vi "Demo1_Filter.vi"(11 "input data":fxp<+/-,16,1>) -> (3 "output data":fxp<+/-,16,2>)   [LabVIEW 2023]
doc: "----------------------\n\nThis filter is configured as follows:\n\n<b>Filter Configuration</b>\nType: Single Rate\nStructure: FIR Direct Form\n\n<b>Input Data Type</b>\nType: fixed-point <±,16,1> [-1.000000E+0,9.999695E-1]:3.051758E-5\n\n<b>Output Data Type</b>\nType: fixed-point <±,16,2> [-2.000000E+0,1.999939E+0]:6.103516E-5\nRounding mode: Truncate\nOverflow mode: Wrap\n\n<b>Implementation</b>\nNumber of channels: 1\nMaximum input sampling rate per channel @ 40MHz: 754.717kHz\nGain processing: On Target\nMethod: Multiple Multiply-Accumulator\nNumber of multiply pipeline stages: 1\n\n<b>Execution Mode</b>\nOutside single-cycle Timed Loop\nThroughput: 53 cycles/sample\n\n<b>Estimated Resources</b>\nNumber of multiply-accumulate units: 1\nMultiply operation: 16bits x 16bits => 32bits"
uses:
  <vilib>/Platform/TimedLoop/XDataNode/timing_clust.ctl
  <vilib>/Platform/TimedLoop/XDataNode/nitl_modes.ctl
  <vilib>/Platform/TimedLoop/XDataNode/wakeup.ctl
  <vilib>/Platform/TimedLoop/XDataNode/XDataNode.xnode
  <vilib>/Platform/TimedLoop/XDataNode/XDNodeRunTimeDep.lvlib
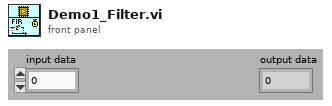
[diagram p1: front panel]
types:
  T1 = typedef "XDNodeRunTimeDep.lvlib/timing_clust.ctl" = cluster{"Expected End [f-1]":u64, "Actual End [f-1]":u64, "Finished Late? [f-1]":bool, "Expected End [i-1]":u64, "Actual End [i-1]":u64, "Finished Late? [i-1]":bool, "Expected Start [i]":u64, "Actual Start [i]":u64, "Expected Start [f]":u64, "Actual Start [f]":u64, "Source Name":string, "Structure Name":string, "Period":i64, "Deadline":i64, "Offset":i64, "Start":i64, "Priority":i32, "Timeout":i32, "Mode":T2, "Wakeup Reason":T3, "Error":errorcluster, "Source Type":string, "Secondary Source Type":string, "Global End Time":u64, "Global Start Time":u64, "Frame Duration":u64, "Iteration Duration":u64, "Assigned CPU":i32, "I/O Scan Engine Mode":u32}
  T2 = typedef "XDNodeRunTimeDep.lvlib/nitl_modes.ctl" = enum32{"No Change", "Process missed periods, maintain original phase", "Discard missed periods, maintain original phase", "Process missed periods, ignore original phase", "Discard missed periods, ignore original phase"}
  T3 = typedef "XDNodeRunTimeDep.lvlib/wakeup.ctl" = enum32{"Normal", "Aborted", "Asynchronous wakeup", "Timing source error", "Timed loop error", "Timeout"}
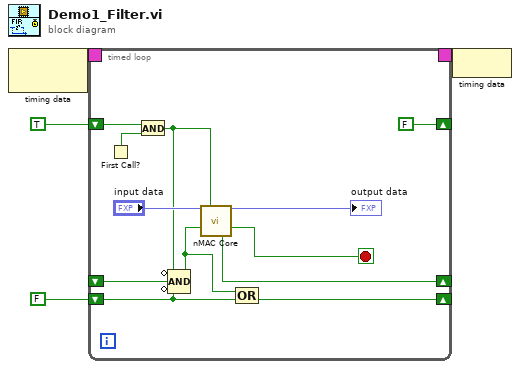
[diagram p0: block diagram]
diagram:
  n1 = node-c288() -> (w2:T1)  [unwired: 1 in]
  n2 = timed-loop "Main Loop" {
    shift-right: [w5] -> _
    shift-left: FALSE -> [w6]
    shift-right: [FALSE] -> _
    shift-left: TRUE -> [w13]
    shift-right: [w8] -> _
    shift-left: _ -> [w9]
    timing: w2 -> [_]
    timing-out: [_] -> w1
    stop <- w14 stop-if-true
    n3 = First Call?() -> (First Call?: T/F=w12:bool)
    n4 = And(x=w13, y=w12) -> (x .and. y?=w10:bool)
    n5 = Compound Arithmetic op=AND(invert w10, w9, invert w6) -> (w7:bool)
    n6 = call "nMAC Core"("input data"="input data", "reset"=w10, "input valid"=w7) -> ("output data"=→"output data":fxp<+/-,16,2>, "output valid"=w14:bool, "ready for input"=w8:bool)  [unwired: 10 in]
    n7 = Compound Arithmetic op=OR(w7, w6) -> (w5:bool)
  }
  n8 = node-c288(w1) -> ()
